vi "SearchStringArray.vi"(10 "stringArray":string[](array[string]), 11 "String":string) -> (3 "foundIndex":i32)   [LabVIEW 2016]
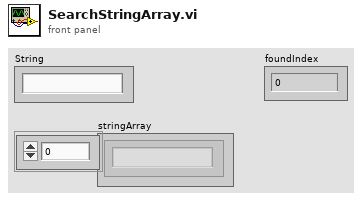
[diagram p1: front panel]
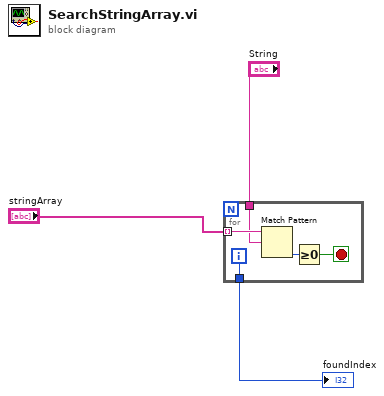
[diagram p0: block diagram]
diagram:
  n1 = for {
    tunnel: "stringArray" -> [w8] mode=indexing
    tunnel: [w5] -> w1
    tunnel: "String" -> [w4]
    i -> [w5]
    stop <- w6 stop-if-true
    n2 = Match Pattern(string=w8, regular expression=w4) -> (offset past match=w7:i32)  [unwired: 1 in, 3 out]
    n3 = Greater Or Equal To 0?(x=w7) -> (x >= 0?=w6:bool)
  }
  "foundIndex" <- w1
